vi "drivable paths global.vi"() -> ()   [LabVIEW 2010]
panel:
  in  "line  raw serial port data":u8
  out "driveable path lengths (lines)":u16[](array[numeric])
  out "driveable path lengths":u16[](array[numeric])
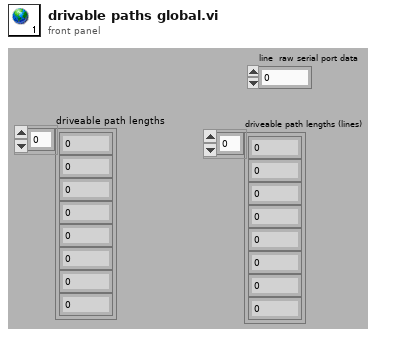
[diagram p1: front panel]
diagram:
